vi "Destroy.vi"(8 "error in (no error)":errorcluster, 11 "ImageRectifier in":refnum<class "ImageDistorter.lvclass">) -> (0 "error out":errorcluster)   [LabVIEW 2020, in "g_ar_toolkit.image.lvlib" / "ImageDistorter.lvclass"]
uses:
  ImageDistorter.lvclass
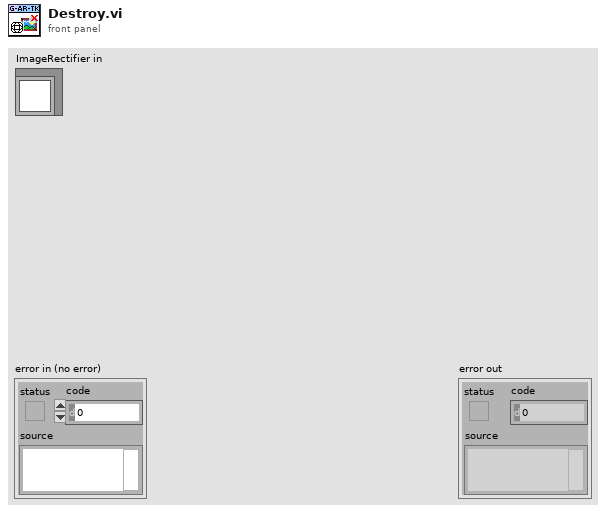
[diagram p1: front panel]
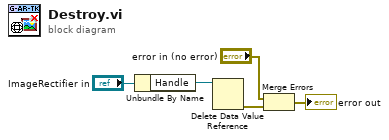
[diagram p0: block diagram]
diagram:
  n1 = Unbundle By Name("ImageRectifier in") -> ("Handle"=w3:refnum<data-value>)
  n2 = Delete Data Value Reference(data value reference=w3) -> (error out=w1:errorcluster)  [unwired: 1 in, 1 out]
  n3 = Merge Errors("error in (no error)", w1) -> (→"error out":errorcluster)
